vi "Convert Radian or Degrees.vi"(7 "Mode":enum16{"To Radians", "To Degrees"}(ring), 8 "AngleIn 4":dbl format="%.4f", 9 "AngleIn 3":dbl format="%.4f", 10 "AngleIn 2":dbl format="%.4f", 11 "AngleIn 1":dbl format="%.4f") -> (0 "AngleOut 4":dbl format="%.4f", 1 "AngleOut 3":dbl format="%.4f", 2 "AngleOut 2":dbl format="%.4f", 3 "AngleOut 1":dbl format="%.4f")   [LabVIEW 2013]
doc: "Converts the four input angles 'AngleIn 1' through 'AngleIn 4' from degrees to radians or vice versa and passes the converted angle out via connectors 'AngleOut 1' through 'AngleOut 4'. The convert mode is set by 'Mode', either \"To Radians\" (the default) or \"To Degrees\".\n\nAutoCon, 7/2000"
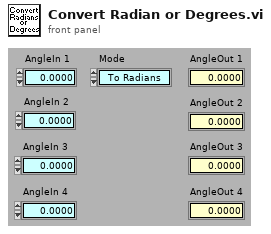
[diagram p1: front panel]
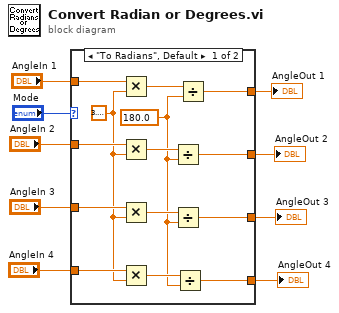
[diagram p0: block diagram]
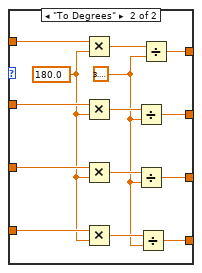
[diagram p2: hidden frame]
diagram:
  n1 = case shown="\"To Radians\", Default" "Mode" {
    tunnel: "AngleIn 1" -> [w23 w37]
    tunnel: "AngleIn 2" -> [w22 w36]
    tunnel: "AngleIn 3" -> [w21 w35]
    tunnel: "AngleIn 4" -> [w20 w34]
    tunnel: [w13 w29] -> w4
    tunnel: [w12 w28] -> w3
    tunnel: [w11 w27] -> w2
    tunnel: [w10 w26] -> w1
    frame "To Radians", Default {
      w14 = 180.0 ("y")
      w19 = 3.141592653589793
      n2 = Multiply(x=w23, y=w19) -> (x*y=w18:dbl)
      n3 = Multiply(x=w22, y=w19) -> (x*y=w17:dbl)
      n4 = Multiply(x=w21, y=w19) -> (x*y=w16:dbl)
      n5 = Multiply(x=w20, y=w19) -> (x*y=w15:dbl)
      n6 = Divide(x=w17, y=w14) -> (x/y=w12:dbl)
      n7 = Divide(x=w16, y=w14) -> (x/y=w11:dbl)
      n8 = Divide(x=w15, y=w14) -> (x/y=w10:dbl)
      n9 = Divide(x=w18, y=w14) -> (x/y=w13:dbl)
    }
    frame "To Degrees" {
      w25 = 180.0 ("y")
      w24 = 3.141592653589793
      n10 = Multiply(x=w37, y=w25) -> (x*y=w33:dbl)
      n11 = Multiply(x=w36, y=w25) -> (x*y=w32:dbl)
      n12 = Multiply(x=w35, y=w25) -> (x*y=w31:dbl)
      n13 = Multiply(x=w34, y=w25) -> (x*y=w30:dbl)
      n14 = Divide(x=w32, y=w24) -> (x/y=w28:dbl)
      n15 = Divide(x=w31, y=w24) -> (x/y=w27:dbl)
      n16 = Divide(x=w30, y=w24) -> (x/y=w26:dbl)
      n17 = Divide(x=w33, y=w24) -> (x/y=w29:dbl)
    }
  }
  "AngleOut 1" <- w4
  "AngleOut 2" <- w3
  "AngleOut 3" <- w2
  "AngleOut 4" <- w1
